vi "x-y curves and z data to three-column data.vi"(10 "z label values":dbl[](array[numeric]), 11 "x-y curves":cluster{dbl[], dbl[]}[](array[cluster])) -> (1 "z":dbl[](array[numeric]), 2 "y":dbl[](array[numeric]), 3 "x":dbl[](array[numeric]))   [LabVIEW 2020]
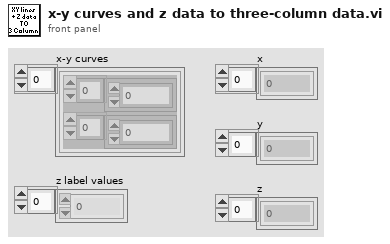
[diagram p1: front panel]
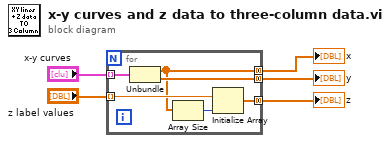
[diagram p0: block diagram]
diagram:
  n1 = for {
    tunnel: "x-y curves" -> [w11] mode=indexing
    tunnel: [w6] -> w3 mode=concatenating
    tunnel: [w8] -> w4 mode=concatenating
    tunnel: "z label values" -> [w10] mode=indexing
    tunnel: [w7] -> w5 mode=concatenating
    n2 = Unbundle(w11) -> (w6:dbl[], w8:dbl[])
    n3 = Array Size(array=w6) -> (size(s)=w9:i32)
    n4 = Initialize Array(w10, w9) -> (w7:dbl[])
  }
  "z" <- w5
  "y" <- w4
  "x" <- w3
